vi "Backsave LabVIEW File.vi"(8 "Error In":errorcluster, 9 "LabVIEW Version":T1, 10 "Destination Path":path, 11 "LabVIEW File":path) -> (0 "Error Out":errorcluster, 2 "Warnings":string)   [LabVIEW 2020, in "LMH-Toolbox.lvlib"]
uses:
  LMH-Toolbox.lvlib
  Private/Type Defs/LabVIEW Version.ctl
  Private/VI Tools/LMH-VITools.lvlib
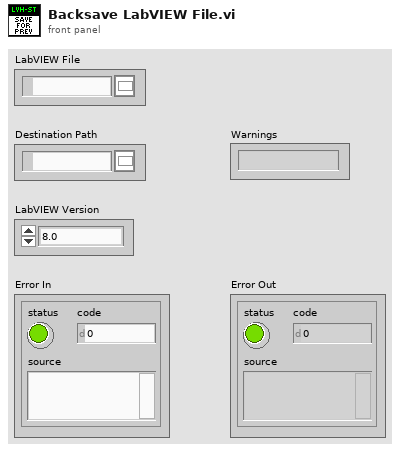
[diagram p1: front panel]
types:
  T1 = typedef "LMH-Toolbox.lvlib/LabVIEW Version.ctl" = enum16{"8.0", "8.2", "8.6", "9.0", "10.0", "11.0", "12.0", "13.0"}
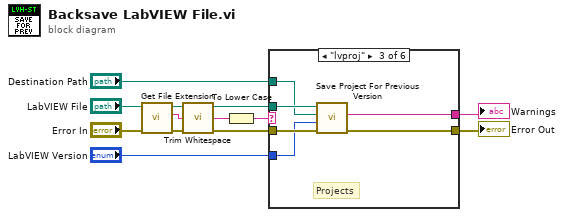
[diagram p0: block diagram]
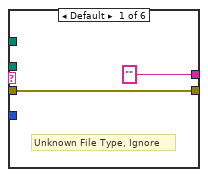
[diagram p2: hidden frame]
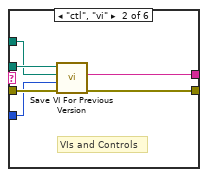
[diagram p3: hidden frame]
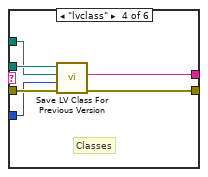
[diagram p4: hidden frame]
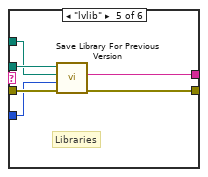
[diagram p5: hidden frame]
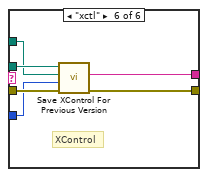
[diagram p6: hidden frame]
diagram:
  n1 = call "Get File Extension.vi"("Error In"="Error In", "File Path Control"="LabVIEW File") -> ("Error Out"=w9:errorcluster, "Extension"=w8:string, "Duplicate Path"=w5:path)  [unwired: 7 in]
  n2 = call <vilib>:"Trim Whitespace.vi"("string"=w8) -> ("trimmed string"=w7:string)  [unwired: 1 in]
  n3 = To Lower Case(string=w7) -> (all lower case string=w6:string)
  n4 = case shown="\"lvproj\"" w6 {
    tunnel: w9 -> [w12 w18 w25 w31 w36 w42]
    tunnel: w5 -> [_ w19 w24 w30 w37 w40]
    tunnel: "Destination Path" -> [_ w17 w23 w29 w35 w39]
    tunnel: "LabVIEW Version" -> [_ w16 w22 w28 w34 w38]
    tunnel: [w12 w15 w20 w27 w33 w43] -> w2
    tunnel: ["" ("Warnings") w14 w21 w26 w32 w41] -> w1
    frame Default {
      # "Unknown File Type, Ignore"
    }
    frame "ctl", "vi" {
      # "VIs and Controls"
      n5 = call "Save VI For Previous Version.vi"("Error In"=w18, "LabVIEW Version"=w16, "Save Path"=w17, "VI Path"=w19) -> ("Error Out"=w15:errorcluster, "Warnings"=w14:string)  [unwired: 6 in]
    }
    frame "lvproj" {
      # "Projects"
      n6 = call "Save Project For Previous Version.vi"("Error In"=w25, "LabVIEW Version"=w22, "Save Directory"=w23, "Project Path"=w24) -> ("Error Out"=w20:errorcluster, "Warnings"=w21:string)  [unwired: 6 in]
    }
    frame "lvclass" {
      # "Classes"
      n7 = call "Save LV Class For Previous Version.vi"("Error In"=w31, "LabVIEW Version"=w28, "Save Path"=w29, "Class Path"=w30) -> ("Error Out"=w27:errorcluster, "Warnings"=w26:string)  [unwired: 6 in]
    }
    frame "lvlib" {
      # "Libraries"
      n8 = call "Save Library For Previous Version.vi"("Error In"=w36, "LabVIEW Version"=w34, "Save Path"=w35, "Library Path"=w37) -> ("Error Out"=w33:errorcluster, "Warnings"=w32:string)  [unwired: 6 in]
    }
    frame "xctl" {
      # "XControl"
      n9 = call "Save XControl For Previous Version.vi"("Error In"=w42, "LabVIEW Version"=w38, "Save Path"=w39, "XControl Path"=w40) -> ("Error Out"=w43:errorcluster, "Warnings"=w41:string)  [unwired: 6 in]
    }
  }
  "Error Out" <- w2
  "Warnings" <- w1
